vi "FGV SAE j-1939 Table Data.vi"(6 "Aktion":enum16{"lesen", "schreiben"}(ring), 8 "Fehler (Eingang, kein Fehler)":errorcluster, 10 "Sorting":i32=2, 11 "Referenz (Eingang)":refnum<k21>) -> (0 "Fehler (Ausgang)":errorcluster, 1 "SAE J-1939 Signal-Cluster":T3[](array[typedef]), 2 "SAE J-1939 Signal Text Array unsorted":string[][](array[string]), 3 "SAE J-1939 Signal Table sorted":string[][](array[string]), 4 "Signal IDs Array":T2(array[cluster]), 5 "Sizes":T1, 7 "Sorting out":i32)   [LabVIEW 2020]
uses:
  SAE J-1938 Signal.ctl
  fd4e3c37-ecf9-4d2f-844f-0c05244779dc.vi
  7dec5452-1572-453f-960f-6994b199a709.vi
  <vilib>/Array/Sort 2D Array - Pop Stack.vi
  <vilib>/Array/Sort 2D Array - Push Stack.vi
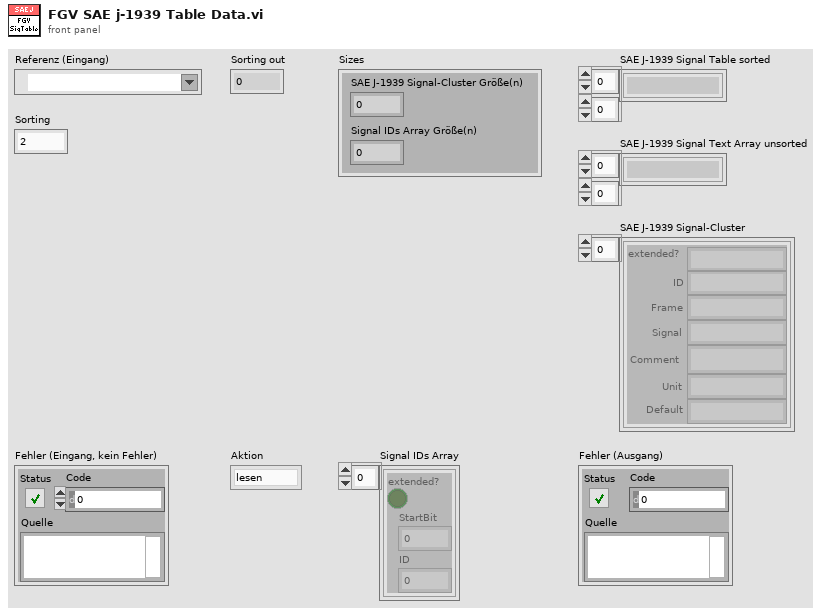
[diagram p1: front panel]
types:
  T1 = cluster{"SAE J-1939 Signal-Cluster Größe(n)":i32, "Signal IDs Array Größe(n)":i32}
  T2 = cluster{"extended?":bool, "StartBit":u32, "ID":u32}[]
  T3 = typedef "OBD Daten.lvlib/SAE J-1938 Signal.ctl" = cluster{"extended?":string, "ID":string, "Frame":string, "Signal":string, "Comment":string, "Unit":string, "Default":string}
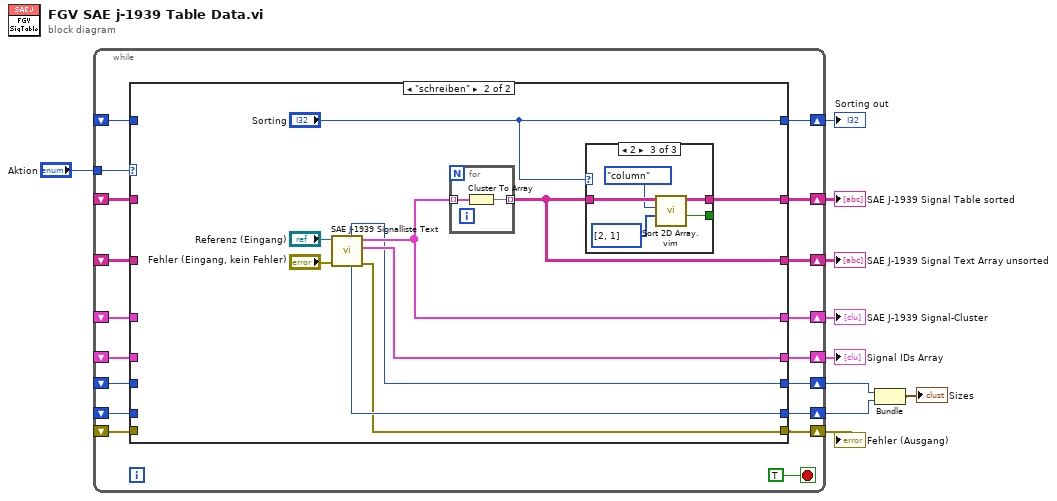
[diagram p0: block diagram]
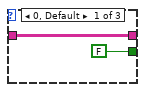
[diagram p3: hidden frame]
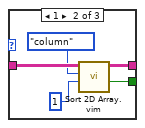
[diagram p4: hidden frame]
diagram:
  n1 = while {
    tunnel: "Aktion" -> [w27]
    shift-right: [w26] -> w9
    shift-left: _ -> [w25]
    shift-right: [w24] -> w8
    shift-left: _ -> [w23]
    shift-right: [w22] -> w7
    shift-left: _ -> [w21]
    shift-right: [w20] -> w6
    shift-left: _ -> [w19]
    shift-right: [w16] -> w5
    shift-left: _ -> [w15]
    shift-right: [w18] -> w3
    shift-left: _ -> [w14]
    shift-right: [w17] -> w2
    shift-left: _ -> [w13]
    shift-right: [w12] -> w4
    shift-left: _ -> [w11]
    stop <- TRUE stop-if-true
    n2 = case shown="\"schreiben\"" w27 {
      tunnel: [w36 w45] -> w26
      tunnel: w25 -> [w36 _]
      tunnel: [w35 w44] -> w24
      tunnel: w23 -> [w35 _]
      tunnel: [w34 w43] -> w22
      tunnel: w21 -> [w34 _]
      tunnel: [w33 w42] -> w20
      tunnel: w19 -> [w33 _]
      tunnel: [w31 w41] -> w18
      tunnel: [w30 w40] -> w17
      tunnel: [w32 w39] -> w16
      tunnel: w15 -> [w32 _]
      tunnel: w14 -> [w31 _]
      tunnel: w13 -> [w30 _]
      tunnel: [w29 "Sorting"] -> w12
      tunnel: w11 -> [w29 _]
      frame "lesen", Default {
      }
      frame "schreiben" {
        n3 = call "SAE J-1939 Signalliste Text.vi"("Fehler (Eingang, kein Fehler)"="Fehler (Eingang, kein Fehler)", "Referenz (Eingang)"="Referenz (Eingang)") -> ("Fehler (Ausgang)"=w39:errorcluster, "Signal IDs Array"=w42:T2, "SAE J-1939 Signal-Cluster"=w43:T3[], "Signal IDs Array Größe(n)"=w40:i32, "SAE J-1939 Signal-Cluster Größe(n)"=w41:i32)  [unwired: 5 in]
        n4 = for {
          tunnel: w43 -> [w60] mode=indexing
          tunnel: [w59] -> w44 mode=indexing
          n5 = Cluster To Array(cluster=w60) -> (array=w59:string[])
        }
        n6 = case shown="2" "Sorting" {
          tunnel: [w48 w52 w57] -> w45
          tunnel: [FALSE ("index out of range?") w51 w56] -> _
          tunnel: w44 -> [w48 w50 w55]
          frame 0, Default {
          }
          frame 1 {
            n7 = call "Sort 2D Array.vim"("index"=1, "dimension to index (column)"=enum16{"column", "row"}."column", "2D array"=w50) -> ("index out of range?"=w51:bool, "sorted 2D array"=w52:string[][])  [unwired: 7 in]
          }
          frame 2 {
            n8 = call "Sort 2D Array.vim"("index"=i32[] [2, 1], "dimension to index (column)"=enum16{"column", "row"}."column", "2D array"=w55) -> ("index out of range?"=w56:bool, "sorted 2D array"=w57:string[][])  [unwired: 7 in]
          }
        }
      }
    }
  }
  "SAE J-1939 Signal Table sorted" <- w9
  "SAE J-1939 Signal Text Array unsorted" <- w8
  "SAE J-1939 Signal-Cluster" <- w7
  "Signal IDs Array" <- w6
  "Fehler (Ausgang)" <- w5
  "Sorting out" <- w4
  n9 = Bundle("SAE J-1939 Signal-Cluster Größe(n)"=w3, "Signal IDs Array Größe(n)"=w2) -> (→"Sizes":T1)  [unwired: 1 in]
